vi "fit -- function controller V2.vi"(7 "fit using":T1=enum."varshni", 9 "y":dbl[](array[numeric]), 10 "x":dbl[](array[numeric])) -> (3 "best fit parameters":dbl[](array[numeric])=[1510.033618014085, -0.06734487332989668, -59.94387240978006])   [LabVIEW 2012]
uses:
  fit function selector control.ctl
  array -- fit control .ctl
  <vilib>/gmath/NumericalOptimization/Nonlinear Curve Fit LM.vi
  <vilib>/gmath/NI_Gmath.lvlib
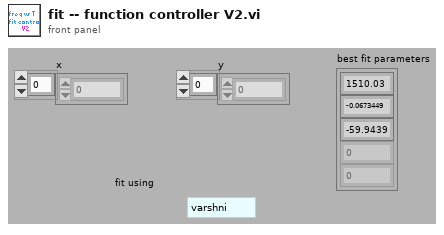
[diagram p1: front panel]
types:
  T1 = typedef "fit function selector control.ctl" = enum16{"linear", "varshni", "varshni5", "LogMinusT", "hyperbola", "einstein", "sine", "sine2theta", "cos2theta"}
  T2 = typedef "array -- fit control .ctl" = enum16{"fit", "calc", "check", "init"}
  T3 = typedef "NI_Gmath.lvlib/LM model function reference.ctl" = refnum<vi>
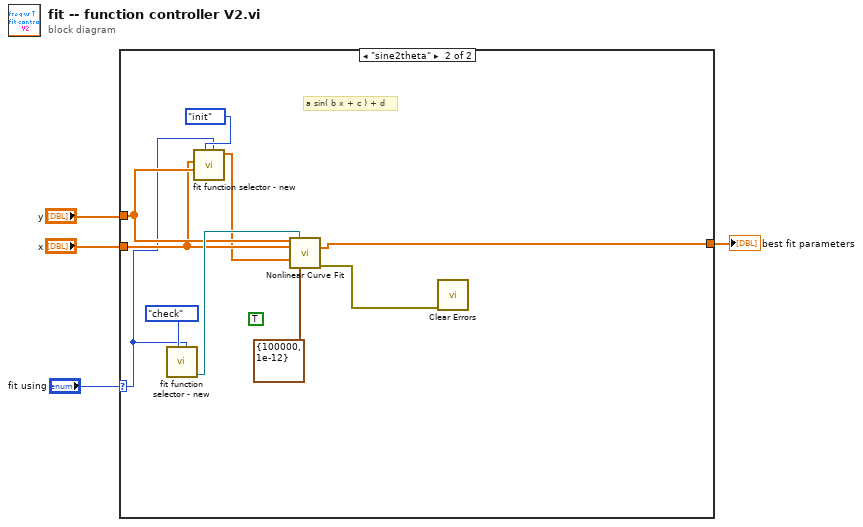
[diagram p0: block diagram]
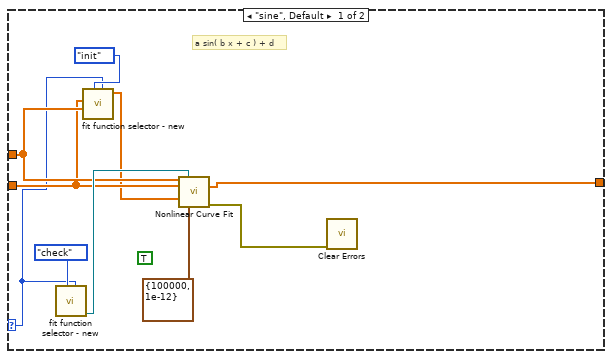
[diagram p2: hidden frame]
diagram:
  n1 = case shown="\"sine2theta\"" "fit using" {
    selector: "fit using" -> [w5 w15]
    tunnel: "y" -> [w9 w19]
    tunnel: "x" -> [w8 w18]
    tunnel: [w12 w22] -> w1
    frame "sine", Default {
      (unwired) TRUE
      # "a sin( b x + c ) + d"
      n2 = call "fit function selector - new.vi"("fit using"=w5, "fit action"=array_--_fit_control_."check") -> ("vi reference"=w10:T3)  [unwired: 5 in, 4 out]
      n3 = call "fit function selector - new.vi"("fit using"=w5, "fit action"=array_--_fit_control_."init", "y"=w9, "x"=w8) -> ("fit params out"=w6:dbl[])  [unwired: 3 in, 4 out]
      n4 = call-poly <vilib>:"Nonlinear Curve Fit.vi"("Y"=w9, "f(x,a)"=w10, "X"=w8, "initial parameters"=w6, "termination"=cluster{"max iteration":i32, "tolerance":dbl} {"max iteration"=100000, "tolerance"=1e-12}) -> ("best fit parameters"=w12:dbl[], "error out"=w13:errorcluster)  [unwired: 5 in, 4 out]
      n5 = call <vilib>:"Clear Errors.vi"("error in (no error)"=w13) -> ()  [unwired: 6 in, 1 out]
    }
    frame "sine2theta" {
      (unwired) TRUE
      # "a sin( b x + c ) + d"
      n6 = call "fit function selector - new.vi"("fit using"=w15, "fit action"=array_--_fit_control_."check") -> ("vi reference"=w20:T3)  [unwired: 5 in, 4 out]
      n7 = call "fit function selector - new.vi"("fit using"=w15, "fit action"=array_--_fit_control_."init", "y"=w19, "x"=w18) -> ("fit params out"=w16:dbl[])  [unwired: 3 in, 4 out]
      n8 = call-poly <vilib>:"Nonlinear Curve Fit.vi"("Y"=w19, "f(x,a)"=w20, "X"=w18, "initial parameters"=w16, "termination"=cluster{"max iteration":i32, "tolerance":dbl} {"max iteration"=100000, "tolerance"=1e-12}) -> ("best fit parameters"=w22:dbl[], "error out"=w23:errorcluster)  [unwired: 5 in, 4 out]
      n9 = call <vilib>:"Clear Errors.vi"("error in (no error)"=w23) -> ()  [unwired: 6 in, 1 out]
    }
  }
  "best fit parameters" <- w1
